vi "FPGA Read.vi"(7 "error in (no error)":errorcluster, 10 "FPGA VI Reference In":refnum<k20>) -> (0 "error out":errorcluster, 2 "FPGA State":enum16{"Normal Operation", "Safe State"}(ring), 3 "FPGA VI Reference Out":refnum<k20>)   [LabVIEW 2011]
uses:
  <vilib>/Utility/error.llb/Error Cluster From Error Code.vi
  <vilib>/rvi/errors/niLvFpgaAdjustHostInterfaceError.vi
  <vilib>/rvi/interface/nirviReadWriteControl/nirviReadWriteControl.xnode
  NiFpgaLv.dll
  <vilib>/rvi/interface/Simulation/niFpgaSimulationCallBeginRW.vi
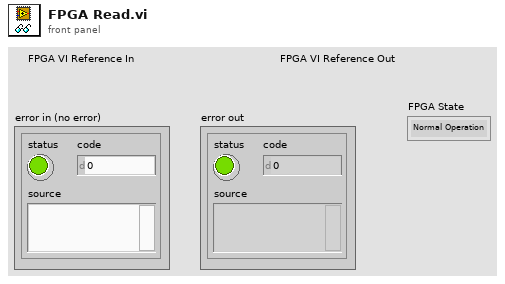
[diagram p1: front panel]
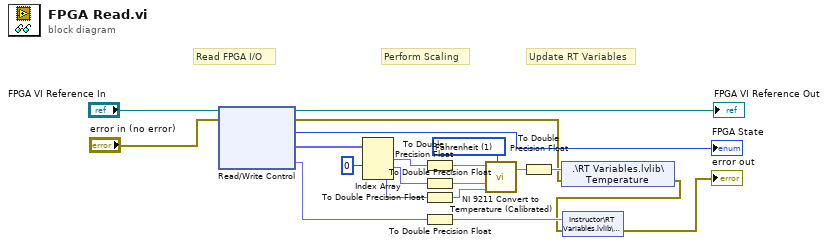
[diagram p0: block diagram]
diagram:
  w15 = u16 1 items=["Celsius", "Fahrenheit", "Kelvin", "Rankine"] ("Temperature Units (C)")
  # "Update RT Variables"
  # "Perform Scaling"
  # "Read FPGA I/O"
  n1 = xnode "Read/Write Control"("FPGA VI Reference In"="FPGA VI Reference In", "error in"="error in (no error)") -> ("FPGA VI Reference Out"=→"FPGA VI Reference Out":refnum<k20>, "error out"=w3:errorcluster, "FPGA State"=→"FPGA State":enum16{"Normal Operation", "Safe State"}, "Temp Data"=w11:fxp<+/-,24,-2>[], "pH"=w5:fxp<+/-,20,5>)
  n2 = Index Array(array=w11, index #1=0 ("index")) -> (element #1=w10:fxp<+/-,24,-2>, element #2=w9:fxp<+/-,24,-2>, element #3=w8:fxp<+/-,24,-2>)  [unwired: 2 in]
  n3 = To Double Precision Float(number=w10) -> (double precision float=w17:dbl)
  n4 = To Double Precision Float(number=w9) -> (double precision float=w18:dbl)
  n5 = To Double Precision Float(number=w8) -> (double precision float=w6:dbl)
  n6 = To Double Precision Float(number=w5) -> (double precision float=w4:dbl)
  n7 = call "NI 9211 Convert to Temperature (Calibrated).vi"("Temperature Units (C)"=w15, "Autozero Channel"=w6, "CJC Channel"=w18, "Thermocouple Channel"=w17) -> ("Linearized Temperature"=w13:sgl)  [unwired: 3 in]
  n8 = To Double Precision Float(number=w13) -> (double precision float=w14:dbl)
  n9 = shared-variable ".\\RT Variables.lvlib\\Temperature"(w14, error in=w3) -> (error out=w2:errorcluster)
  n10 = shared-variable "Instructor\\RT Variables.lvlib\\pH"(w4, error in=w2) -> (error out=→"error out":errorcluster)
